vi "DropVI_PacketTracer_Instance.vi"() -> ()   [LabVIEW 2013]
uses:
  PacketTracer/PacketTracer.lvclass
panel:
  in  "PacketTracer":refnum<class "PacketTracer.lvclass">
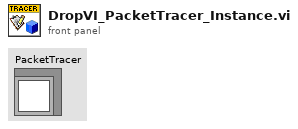
[diagram p1: front panel]
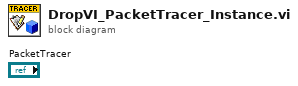
[diagram p0: block diagram]
diagram:
